vi "Propagation.vi"() -> ()   [LabVIEW 2020]
uses:
  StatisticsData.ctl
  HasoSlopes.lvclass
  Pupil.lvclass
  ComputePhaseSet.lvclass
  WavefrontReconstructionMode.ctl
  Phase.lvclass
  HasoField.lvclass
  SurfaceFloat.lvclass
  General dimensions definition.ctl
  Point2D.ctl
  Point2Df.ctl
  HasoData.lvclass
panel:
  out "PSF values":sgl[][](graph)
  in  "Slopes file name":string="Data\\data_phase_computation.has"
  in  "Haso configuration file name":string="Data\\config_file_haso.dat"
  out "PSF Statistics":T1
  out "error out":errorcluster
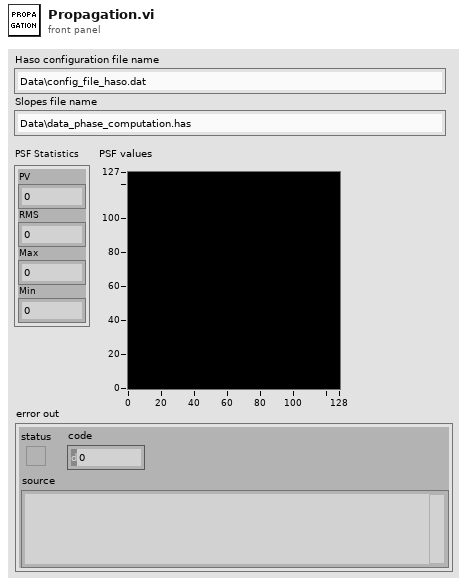
[diagram p1: front panel]
types:
  T1 = typedef "StatisticsData.ctl" = cluster{"PV":sgl, "RMS":dbl, "Max":sgl, "Min":sgl}
  T2 = typedef "General dimensions definition.ctl" = cluster{"Size":T3, "Step":T4}
  T3 = typedef "Point2D.ctl" = cluster{"X":u32, "Y":u32}
  T4 = typedef "Point2Df.ctl" = cluster{"X":sgl, "Y":sgl}
  T5 = cluster{"null_phase":bool, "flat_intensity":bool}
  T6 = typedef "WavefrontReconstructionMode.ctl" = enum16{"None", "Modal_Legendre", "Modal_Zernike", "Zonal", "Modal_Zonal_Zernike", "Modal_Zonal_Legendre"}
  T7 = cluster{"tiltX_mrad":sgl, "tiltY_mrad":dbl, "radius_mm":sgl, "focus_Xpos_mm":sgl, "focus_Ypos_mm":sgl, "astig_angle_rad":sgl, "sagittal_focal_length_mm":sgl, "tangential_focal_length_mm":sgl}
  T8 = typedef "DataHaso acquisition information.ctl" = cluster{"HASO information":T9, "Acquisition information":T10, "SLOPES ENGINE information":T14, "Source wavelength (nm)":dbl, "FillPercent_%":dbl, "session_name":string}
  T9 = typedef "HASO information.ctl" = cluster{"HASO serial number":string, "HASO model":string, "Lower calibration wavelength (nm)":dbl, "Upper calibration wavelength (nm)":dbl, "Revision":i32}
  T10 = typedef "Image information.ctl" = cluster{"Image general information":T11, "Acquisition information":T12, "Number of pixels":T3, "Number of bits":T13}
  T11 = typedef "Image general information.ctl" = cluster{"Camera serial number":string, "Smearing removed":bool, "Background image removed":bool, "Time Stamp":timestamp, "Comment":string, "Camera_MAX_Level":i32}
  T12 = typedef "Image acquisition information.ctl" = cluster{"Exposure duration (us)":i32, "Exposure duration specified (us)":i32, "Gain":sgl, "Number of summed images":i32, "Trigger type":string}
  T13 = typedef "Data alignment enum.ctl" = enum16{"8", "16", "32"}
  T14 = typedef "SlopesEngineSetup.ctl" = cluster{"Start sub-aperture":T3, "Pupil average":dbl}
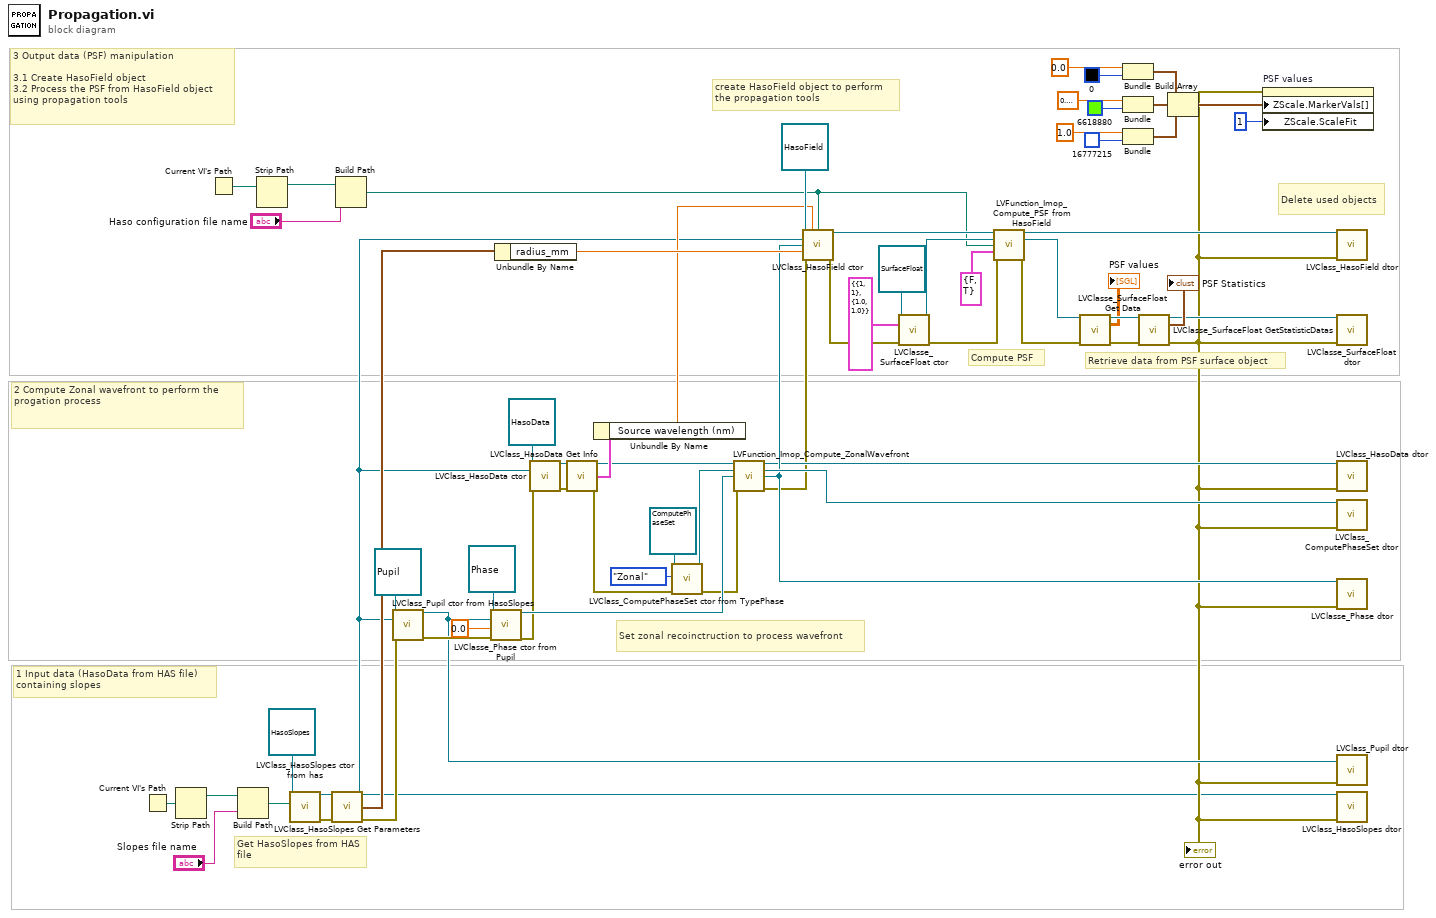
[diagram p0: block diagram]
diagram:
  # "Delete used objects"
  # "Retrieve data from PSF surface object"
  # "Compute PSF"
  # "Set zonal recoinctruction to process wavefront"
  # "3 Output data (PSF) manipulation\n\n3.1 Create HasoField object\n3.2 Process the PSF from HasoField object\nusing propagation tools"
  # "2 Compute Zonal wavefront to perform the\nprogation process"
  # "1 Input data (HasoData from HAS file)\ncontaining slopes"
  # "create HasoField object to perform\nthe propagation tools"
  # "Get HasoSlopes from HAS file"
  n1 = Current VI's Path() -> (path=w47:path)
  n2 = Strip Path(path=w47) -> (stripped path=w42:path)  [unwired: 1 out]
  n3 = Current VI's Path() -> (path=w44:path)
  n4 = Build Path(base path=w42, name or relative path="Slopes file name") -> (appended path=w23:path)
  n5 = Strip Path(path=w44) -> (stripped path=w43:path)  [unwired: 1 out]
  n6 = call "LVClass_HasoSlopes ctor from has.vi"("HasoSlopes in"=refnum<class "HasoSlopes.lvclass"> refnum, ".has path"=w23) -> ("HasoSlopes out"=w8:refnum<class "HasoSlopes.lvclass">, "error out"=w10:errorcluster)  [unwired: 12 in]
  n7 = call "LVClass_HasoSlopes Get Parameters.vi"("HasoSlopes in"=w8, "error in (no error)"=w10) -> ("HasoSlopes out"=w1:refnum<class "HasoSlopes.lvclass">, "Pamameter"=w7:T7, "error out"=w9:errorcluster)  [unwired: 11 in]
  n8 = Build Path(base path=w43, name or relative path="Haso configuration file name") -> (appended path=w11:path)
  n9 = call "LVClass_Pupil ctor from HasoSlopes.vi"("Pupil in"=refnum<class "Pupil.lvclass"> refnum, "HasoSlopes.lvclass"=w1, "error in (no error)"=w9) -> ("Pupil out"=w19:refnum<class "Pupil.lvclass">, "error out"=w59:errorcluster)  [unwired: 11 in]
  n10 = call "LVClasse_Phase ctor from Pupil.vi"("Phase in"=refnum<class "Phase.lvclass"> refnum, "Pupil"=w19, "coef"=sgl 0.0, "error in (no error)"=w59) -> ("Phase out"=w26:refnum<class "Phase.lvclass">, "error out"=w21:errorcluster)  [unwired: 10 in]
  n11 = Unbundle By Name(w7) -> ("radius_mm"=w41:sgl)
  n12 = call "LVClass_HasoData ctor.vi"("HasoData in"=refnum<class "HasoData.lvclass"> refnum, "HasoSlopes.lvclass"=w1, "error in (no error)"=w21) -> ("HasoData out"=w15:refnum<class "HasoData.lvclass">, "error out"=w18:errorcluster)  [unwired: 11 in]
  n13 = call "LVClass_HasoData Get Info.vi"("HasoData in"=w15, "error in (no error)"=w18) -> ("HasoData out"=w14:refnum<class "HasoData.lvclass">, "DataHaso acquisition information 2"=w17:T8)  [unwired: 11 in, 1 out]
  n14 = Unbundle By Name(w17) -> ("Source wavelength (nm)"=w12:dbl)
  n15 = call "LVClass_ComputePhaseSet ctor from TypePhase.vi"("ComputePhaseSet in"=refnum<class "ComputePhaseSet.lvclass"> refnum, "TypePhase"=WavefrontReconstructionMode."Zonal", "error in (no error)"=w18) -> ("ComputePhaseSet out"=w27:refnum<class "ComputePhaseSet.lvclass">, "error out"=w20:errorcluster)  [unwired: 11 in]
  n16 = call "LVFunction_Imop_Compute_ZonalWavefront.vi"("HasoData.lvclass"=w14, "ComputePhaseSet.lvclass"=w27, "Phase"=w26, "error constant"=w20) -> ("HasoData.lvclass (dup)"=w16:refnum<class "HasoData.lvclass">, "ComputePhaseSet.lvclass 2"=w25:refnum<class "ComputePhaseSet.lvclass">, "Phase"=w24:refnum<class "Phase.lvclass">, "error out"=w6:errorcluster)  [unwired: 8 in]
  n17 = call "LVClass_HasoField ctor.vi"("HasoField in"=refnum<class "HasoField.lvclass"> refnum, "wavelenght nm"=w12, "haso_config_file_path"=w11, "HasoSlopes.lvclass"=w1, "Phase.lvclass"=w24, "radius_of_curvature _ mm"=w41, "error in (no error)"=w6) -> ("HasoField out"=w57:refnum<class "HasoField.lvclass">, "error out"=w5:errorcluster)  [unwired: 5 in, 2 out]
  n18 = call "LVClasse_SurfaceFloat ctor.vi"("SurfaceFloat in"=refnum<class "SurfaceFloat.lvclass"> refnum, "Dimensions_um"=T2 {"Size"={"X"=1, "Y"=1}, "Step"={"X"=1.0, "Y"=1.0}} ("Dimensions_µm"), "error in (no error)"=w5) -> ("SurfaceFloat out"=w56:refnum<class "SurfaceFloat.lvclass">, "error out"=w4:errorcluster)  [unwired: 11 in]
  n19 = call "LVFunction_Imop_Compute_PSF from HasoField.vi"("HasoField in"=w57, "Surface PSF"=w56, "Path"=w11, "param"=T5 {"null_phase"=FALSE, "flat_intensity"=TRUE}, "error in (no error)"=w4) -> ("HasoField out"=w13:refnum<class "HasoField.lvclass">, "Surface PSF"=w40:refnum<class "SurfaceFloat.lvclass">, "error out"=w39:errorcluster)  [unwired: 8 in]
  n20 = call "LVClasse_SurfaceFloat Get Data.vi"("SurfaceFloat in"=w40, "error in (no error)"=w39) -> ("SurfaceFloat out"=w51:refnum<class "SurfaceFloat.lvclass">, "data"=→"PSF values":sgl[][], "error out"=w50:errorcluster)  [unwired: 11 in]
  n21 = Bundle(0.0, u32 0) -> (w33:cluster{dbl, u32})  [unwired: 1 in]
  n22 = Bundle(sgl 0.2, u32 6618880) -> (w28:cluster{sgl, u32})  [unwired: 1 in]
  n23 = Bundle(sgl 1.0, u32 16777215) -> (w29:cluster{sgl, u32})  [unwired: 1 in]
  n24 = call "LVClasse_SurfaceFloat GetStatisticDatas.vi"("SurfaceFloat in"=w51, "error in (no error)"=w50) -> ("SurfaceFloat out"=w48:refnum<class "SurfaceFloat.lvclass">, "StatisticsData"=→"PSF Statistics":T1, "error out"=w3:errorcluster)  [unwired: 11 in]
  "error out" <- w3
  n25 = Build Array(w33, w28, w29) -> (w32:cluster{dbl, u32}[])
  n26 = property on="PSF values" class="IntGraph (strict)"(error in=w3, "ZScale.MarkerVals[]"=w32, "ZScale.ScaleFit"=u8 1 ("Z Scale.Scale Fit")) -> ()  [unwired: 1 in, 2 out]
  n27 = call "LVClass_HasoField dtor.vi"("HasoField in"=w13, "error in (no error)"=w3) -> ()  [unwired: 12 in, 2 out]
  n28 = call "LVClasse_SurfaceFloat dtor.vi"("SurfaceFloat in"=w48, "error in (no error)"=w3) -> ()  [unwired: 12 in, 2 out]
  n29 = call "LVClass_HasoData dtor.vi"("HasoData in"=w16, "error in (no error)"=w3) -> ()  [unwired: 12 in, 2 out]
  n30 = call "LVClass_ComputePhaseSet dtor.vi"("ComputePhaseSet in"=w25, "error in (no error)"=w3) -> ()  [unwired: 12 in, 2 out]
  n31 = call "LVClasse_Phase dtor.vi"("Phase in"=w24, "error in (no error)"=w3) -> ()  [unwired: 12 in, 2 out]
  n32 = call "LVClass_Pupil dtor.vi"("Pupil in"=w19, "error in (no error)"=w3) -> ()  [unwired: 12 in, 2 out]
  n33 = call "LVClass_HasoSlopes dtor.vi"("HasoSlopes in"=w1, "error in (no error)"=w3) -> ()  [unwired: 12 in, 2 out]
